vi "InitScope_5160.vi"(5 "Chart length":i32, 6 "Trigger ource":T2, 7 "SCOPE Resource":refnum<k15>="Dev1" caption="NI-Scope Resource", 8 "error in":errorcluster, 9 "input impedance":u32(ring) caption="Input Impedance" items=["1 mega ohm"=0, "50 ohms"=2], 10 "data mode":T1, 11 "FPGA ref":T3) -> (0 "error out":errorcluster, 3 "scope params":T4={"scope mode"=enum."Stopped", "ticker"=refnum, "5160 samples per trigger"=0, "FPGA ref"=refnum, "P2P params"={"instrument handle"="", "stream session"=refnum, "scale"={"offset"=0.0, "gain"=0.0, "reserved 1"=0.0, "reserved 2"=0.0}, "actual sample rate"=10000000.0, "Trigger"=enum."PFI 0", "SCOPE Resource"="Dev1", "input impedance"=0}, "data mode"=enum."Real IO", "5782 samples per record"=0, "Chart length"=0} {"P2P params"."input impedance" items=["1 mega ohm"=0, "50 ohms"=2]; "P2P params"."actual sample rate" format="%.2p"})   [LabVIEW 2013]
uses:
  controls/scope_params.ctl
  Utilities/Ticker/Ticker.lvclass
  controls/ScopeMode.ctl
  Config/FPGAref.ctl
  P2P streaming/P2P params.ctl
  P2P streaming/trigger_source.ctl
  FPGA/DataMode.ctl
  <vilib>/rvi/interface/common/niFpgaWaitOnOcc.vi
  <vilib>/Utility/error.llb/Error Cluster From Error Code.vi
  <vilib>/rvi/errors/niLvFpgaAdjustHostInterfaceError.vi
  <vilib>/rvi/interface/nirviReadWriteControl/nirviReadWriteControl.xnode
  NiFpgaLv.dll
  <vilib>/rvi/interface/Simulation/niFpgaSimulationCallBeginRW.vi
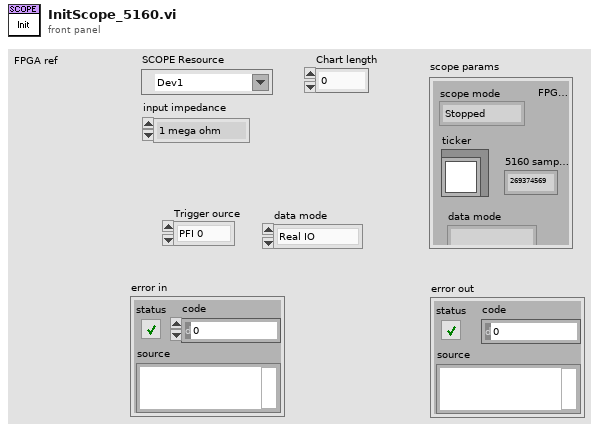
[diagram p1: front panel]
types:
  T1 = typedef "DataMode.ctl" = enum16{"Real IO", "Simulated"}
  T2 = typedef "trigger_source.ctl" = enum16{"PFI 0", "PFI 1", "Software"}
  T3 = typedef "FPGAref.ctl" = refnum<k20>
  T4 = typedef "scope_params.ctl" = cluster{"scope mode":T5, "ticker":refnum<class "Ticker.lvclass">, "5160 samples per trigger":u32, "FPGA ref":T3, "P2P params":T6, "data mode":T1, "5782 samples per record":u32, "Chart length":i32}
  T5 = typedef "ScopeMode.ctl" = enum16{"Stopped", "Single", "Running", "Continuous"}
  T6 = typedef "P2P params.ctl" = cluster{"instrument handle":refnum<k15>, "stream session":refnum<k20>, "scale":cluster{"offset":dbl, "gain":dbl, "reserved 1":dbl, "reserved 2":dbl}, "actual sample rate":dbl, "Trigger":T2, "SCOPE Resource":refnum<k15>, "input impedance":u32}
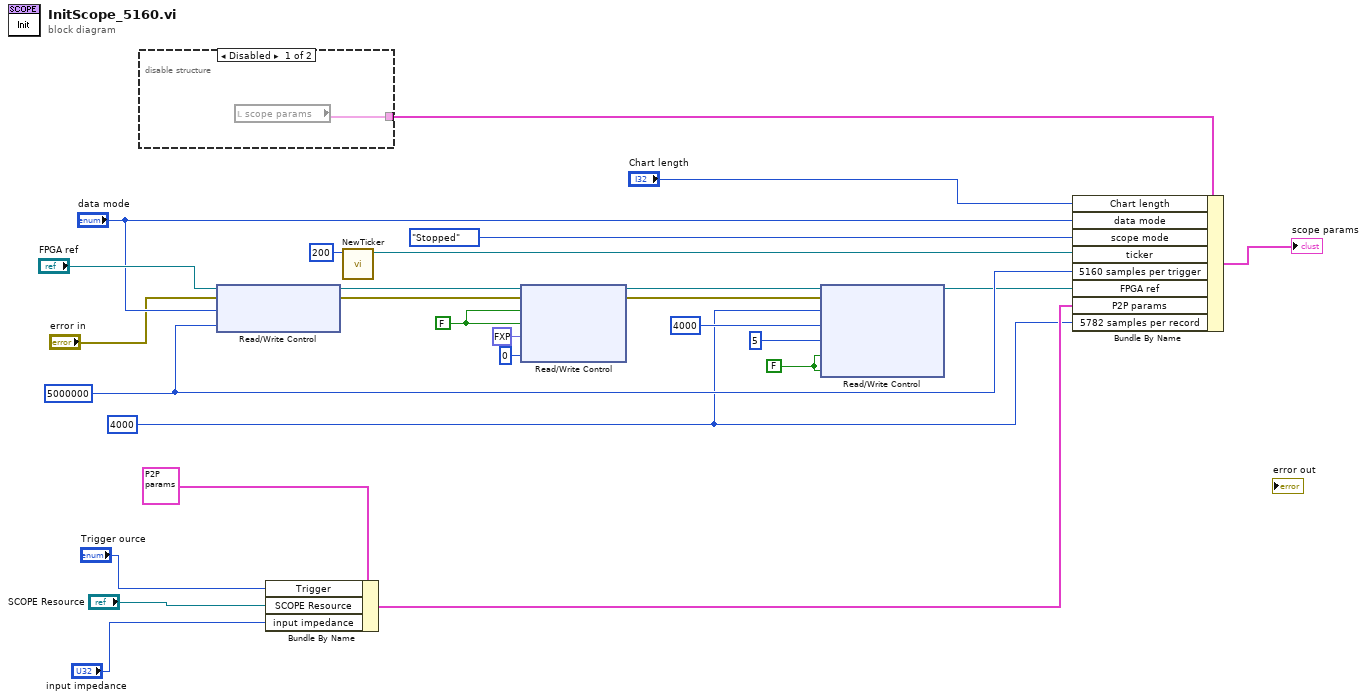
[diagram p0: block diagram]
diagram:
  w2 = u16 4000 ("5782 record length")
  w9 = FALSE
  w10 = FALSE ("Set downsample")
  w15 = 5000000 ("Samples Per Trigger")
  n1 = disable-structure shown="Disabled" {
    disable-tunnel: [w28 _] -> w27
    frame Disabled {
      n2 = local read "scope params"() -> (w28:T4)
    }
    frame Enabled {
    }
  }
  n3 = xnode "Read/Write Control"("FPGA VI Reference In"="FPGA ref", "error in"="error in", "Mode"="data mode", "Samples Per Trigger"=w15) -> ("FPGA VI Reference Out"=w13:T3, "error out"=w4:errorcluster)
  n4 = Bundle By Name(cluster=T6 {"instrument handle"="", "stream session"=refnum, "scale"={"offset"=0.0, "gain"=0.0, "reserved 1"=0.0, "reserved 2"=0.0}, "actual sample rate"=10000000.0, "Trigger"=enum."PFI 0", "SCOPE Resource"="Dev1", "input impedance"=0} ("P2P params"), "Trigger"="Trigger ource", "SCOPE Resource"="SCOPE Resource", "input impedance"="input impedance") -> (w18:T6)
  n5 = call "NewTicker.vi"("Period"=u32 200) -> ("Ticker"=w24:refnum<class "Ticker.lvclass">)  [unwired: 10 in]
  n6 = xnode "Read/Write Control"("FPGA VI Reference In"=w13, "error in"=w4, "new coeffs"=w10, "Set downsample"=w10, "Downsample"=fxp<+,8,8> 0.0, "FIR shift"=0) -> ("FPGA VI Reference Out"=w6:T3, "error out"=w3:errorcluster)
  n7 = xnode "Read/Write Control"("FPGA VI Reference In"=w6, "error in"=w3, "5782 record length"=w2, "quiet time"=u16 4000 ("Samples to aqcuire"), "trigger samples"=u16 5, "Trigger Acquisition"=w9, "Acquisition running"=w9) -> ("FPGA VI Reference Out"=w5:T3)  [unwired: 1 out]
  n8 = Bundle By Name(cluster=w27, "Chart length"="Chart length", "data mode"="data mode", "scope mode"=ScopeMode."Stopped", "ticker"=w24, "5160 samples per trigger"=w15, "FPGA ref"=w5, "P2P params"=w18, "5782 samples per record"=w2) -> (→"scope params":T4)
